vi "RT Loop - Analyze Acceleration_1.vi"(7 "testing":bool, 8 "error in (no error)":errorcluster, 9 "Acceleration RT FIFO In":T1, 10 "FPGA VI Reference Out":refnum<k20>, 11 "Message Queue":refnum<queue>) -> (1 "Acceleration RT FIFO Out":T1)   [LabVIEW 2017]
doc: "Read and analyze acceleration waveform data from FPGA via DMA FIFO. If the acceleration is over the limit, then send the acceleration waveform data to the Log Data Loop."
uses:
  <vilib>/rvi/interface/nirviMethod/nirviMethod.xnode
  <vilib>/FPGAPlugInAG/Dynamic/niLvFpga_ReadFifo_Dynamic.vi
  <vilib>/rvi/errors/niLvFpgaMergeErrorWithErrorCode.vi
  Globals/Global - All RT Loop Stop.vi
  Globals/Global - Configuration Options.vi
  UI Error Handlers/support/Logging/Logging.lvlib
  UI Error Handlers/support/Message Queue/Message Cluster.ctl
  UI Error Handlers/support/Message Queue/Message Queue.lvlib
  controls/Acceleration RT FIFO Reference.ctl
panel:
  out "x-y":u32
  out "G1 status":cluster{"G1 trigger":bool}
  out "G1 status.G1 trigger":bool
  out "sta":bool
  out "logical OR":bool
  in  "Data Rate (Hz)":dbl
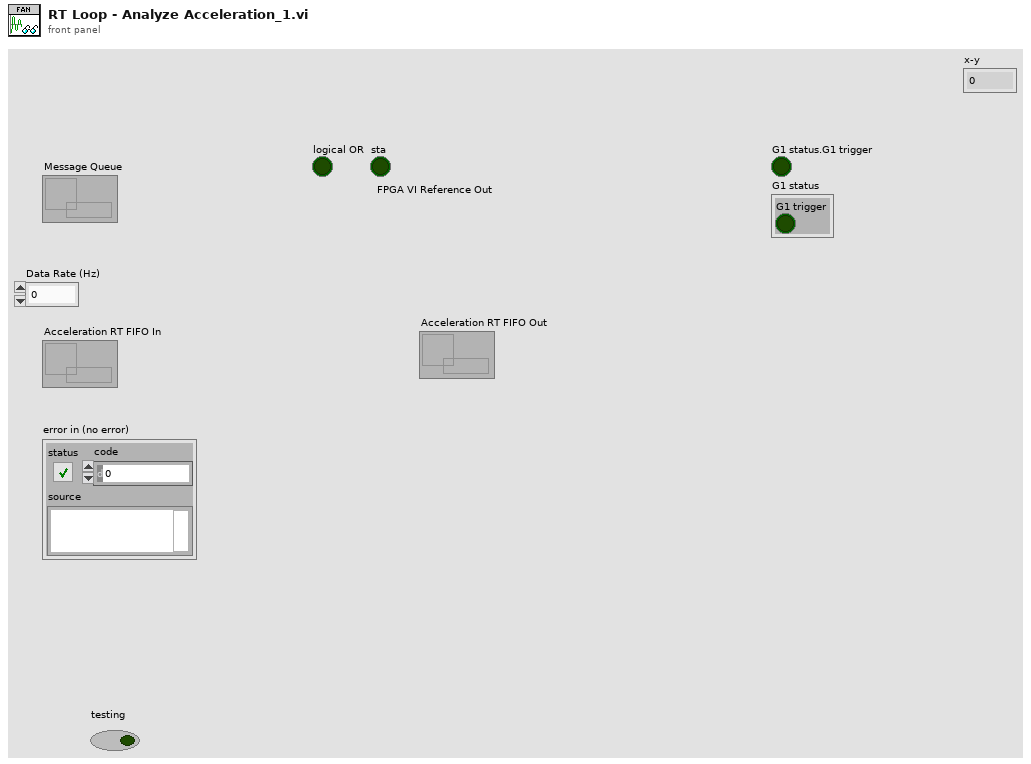
[diagram p1: front panel]
types:
  T1 = typedef "Acceleration RT FIFO Reference.ctl" = refnum<k33>
  T2 = cluster{"Tool data":cluster{"Number of teeth":sgl}, "Cutting data":cluster{"rpm":sgl}, "Limits":cluster{"Magnitude threshold":sgl, "Tolerance":sgl}, "G1 status":cluster{"G1 trigger":bool}}
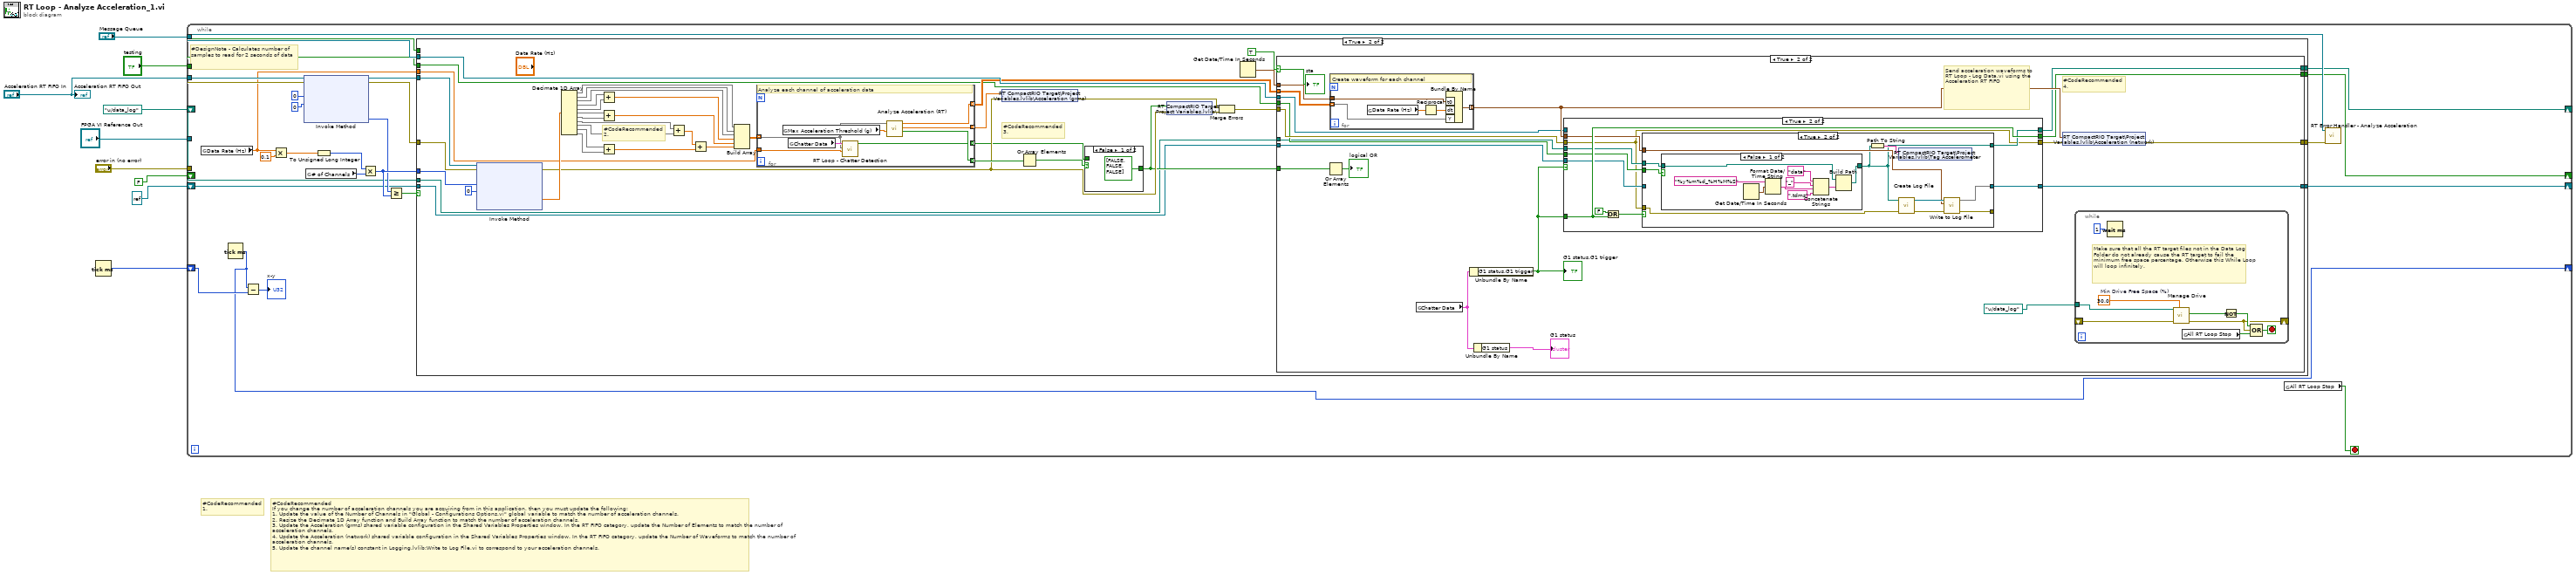
[diagram p0: block diagram]
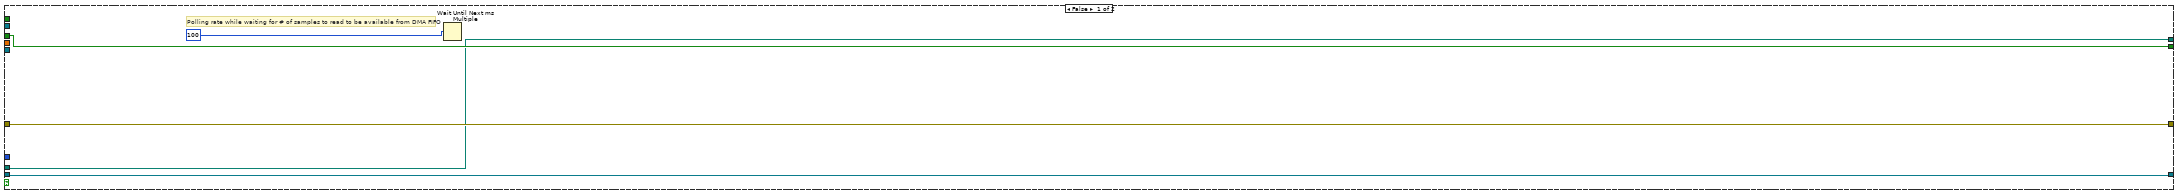
[diagram p2: hidden frame]
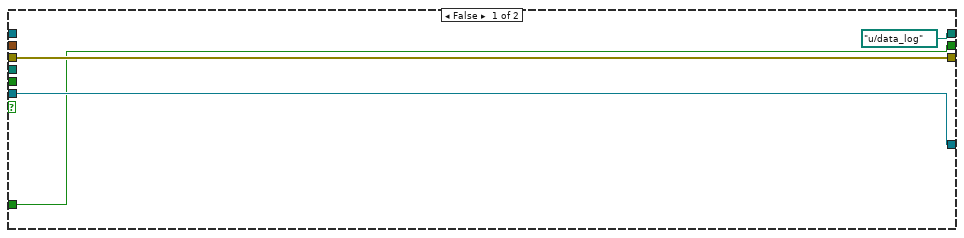
[diagram p5: hidden frame]
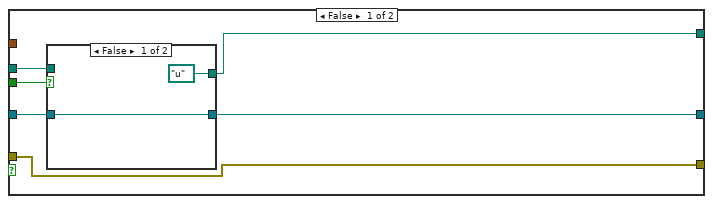
[diagram p6: hidden frame]
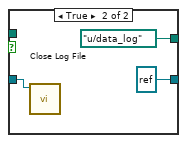
[diagram p7: hidden frame]
diagram:
  # "#CodeRecommended\n1."
  # "#CodeRecommended\nIf you change the number of acceleration channels you are acquiring from in this application, then you must update the following:\n1. Update the value of the Number of Channels in \"Global - Configurations Options.vi\" global variable to match the number of acceleration channels.\n2. Resize the Decimate 1D Array function and Build Array function to match the number of acceleration channels. \n3. Update the Acceleration (grms) shared variable configuration in the Shared Variables Properties window. In the RT FIFO category, update the Number of Elements to match the number of acceleration channels. \n4. Update the Acceleration (network) shared variable configuration in the Shared Variables Properties window. In the RT FIFO category, update the Number of Waveforms to match the number of acceleration channels.\n5. Update the channel name(s) constant in Logging.lvlib:Write to Log File.vi to correspond to your acceleration channels."
  n1 = Tick Count (ms)() -> (millisecond timer value=w1:u32)
  n2 = while {
    tunnel: "FPGA VI Reference Out" -> [w37]
    tunnel: "error in (no error)" -> [w36]
    tunnel: "Message Queue" -> [w29]
    tunnel: "Acceleration RT FIFO In" -> [w27]
    tunnel: "testing" -> [w19]
    shift-right: [w16] -> _
    shift-left: path "u:/data_log" ("AVI Path") -> [w15]
    shift-right: [w18] -> _
    shift-left: FALSE -> [w17]
    shift-right: [w14] -> _
    shift-left: refnum<k34> refnum ("Log File out") -> [w13]
    shift-right: [w11] -> _
    shift-left: w1 -> [w12]
    stop <- w30 stop-if-true
    # "#DesignNote - Calculates number of samples to read for 2 seconds of data"
    n3 = global read "Global - Configuration Options.vi" "Data Rate (Hz)"() -> (w21:dbl)
    n4 = Tick Count (ms)() -> (millisecond timer value=w11:u32)
    n5 = Subtract(x=w11, y=w12) -> (x-y=→"x-y":u32)
    n6 = Multiply(x=w21, y=0.1) -> (x*y=w25:dbl)
    n7 = xnode "Invoke Method"("FPGA VI Reference In"=w37, "error in"=w36, "Number of Elements"=u32 0, "Timeout (ms)"=0) -> ("FPGA VI Reference Out"=w33:refnum<k20>, "error out"=w32:errorcluster, "Elements Remaining"=w20:u32)  [unwired: 1 out]
    n8 = global read "Global - Configuration Options.vi" "# of Channels"() -> (w22:u32)
    n9 = To Unsigned Long Integer(number=w25) -> (unsigned 32bit integer=w24:u32)
    n10 = Multiply(x=w24, y=w22) -> (x*y=w23:u32)
    n11 = Greater Or Equal?(x=w20, y=w23) -> (x >= y?=w31:bool)
    n12 = case shown="True" w31 {
      tunnel: w33 -> [_ w85]
      tunnel: w32 -> [w42 w84]
      tunnel: [w42 w80] -> w28
      tunnel: w23 -> [_ w83]
      tunnel: w27 -> [_ w78]
      tunnel: w21 -> [_ w74]
      tunnel: w19 -> [_ _]
      tunnel: [w40 w66] -> w18
      tunnel: w17 -> [w40 w65]
      tunnel: [w39 w64] -> w16
      tunnel: w15 -> [w39 w63]
      tunnel: [w38 w62] -> w14
      tunnel: w13 -> [w38 w61]
      frame False {
        # "Polling rate while waiting for # of samples to read to be available from DMA FIFO"
        n13 = Wait Until Next ms Multiple(millisecond multiple=u32 100) -> ()  [unwired: 1 out]
      }
      frame True {
        # "#CodeRecommended\n3."
        # "#CodeRecommended\n2."
        n14 = xnode "Invoke Method"("FPGA VI Reference In"=w85, "error in"=w84, "Number of Elements"=w83, "Timeout (ms)"=0) -> ("error out"=w73:errorcluster, "Data"=w77:sgl[])  [unwired: 2 out]
        n15 = Decimate 1D Array(w77) -> (w58:sgl[], w57:sgl[], w56:sgl[], w55:sgl[], w54:sgl[], w52:sgl[], w51:sgl[], w50:sgl[], w49:sgl[], w48:sgl[], w47:sgl[])
        n16 = Add(x=w55, y=w54) -> (x+y=w53:sgl[])
        n17 = Add(x=w52, y=w51) -> (x+y=w43:sgl[])
        n18 = Add(x=w48, y=w47) -> (x+y=w45:sgl[])
        n19 = Add(x=w50, y=w49) -> (x+y=w46:sgl[])
        n20 = Add(x=w46, y=w45) -> (x+y=w44:sgl[])
        n21 = Build Array(w58, w57, w56, w53, w43, w44) -> (w59:sgl[][])
        n22 = for {
          tunnel: [w95] -> w79 mode=indexing
          tunnel: [w94] -> w76 mode=indexing
          tunnel: [w93] -> w75 mode=indexing
          tunnel: w74 -> [w91]
          tunnel: [w90] -> w68 mode=indexing
          tunnel: w59 -> [w88] mode=indexing
          # "Analyze each channel of acceleration data"
          n23 = global read "Global - Configuration Options.vi" "Max Acceleration Threshold (g)"() -> (w92:sgl)
          n24 = global read "Global - Configuration Options.vi" "Chatter Data"() -> (w89:T2)
          n25 = call "RT Loop - Chatter Detection.vi"("Data Rate (Hz)"=w91, "Acceleration Waveform (SGL)"=w88, "Chatter Data"=w89) -> ("Chatter?"=w90:bool)  [unwired: 8 in]
          n26 = call "Analyze Acceleration (RT).vi"("Max Instantaneous Acceleration (g)"=w92, "Acceleration Waveform (SGL)"=w88) -> ("Over Limit?"=w95:bool, "Acceleration (grms)"=w93:dbl, "Acceleration Waveform (DBL)"=w94:dbl[])  [unwired: 7 in]
        }
        n27 = shared-variable "RT CompactRIO Target\\Project Variables.lvlib\\Acceleration (grms)"(w75, error in=w73) -> (error out=w71:errorcluster)
        n28 = Or Array Elements(Boolean array=w79) -> (logical OR=w69:bool)
        n29 = case shown="False" w69 {
          tunnel: w68 -> [_ w87]
          tunnel: [bool[] [FALSE, FALSE, FALSE] ("Chatter?") w87] -> w67
          frame False {
          }
          frame True {
          }
        }
        n30 = shared-variable "RT CompactRIO Target\\Project Variables.lvlib\\Chatter?"(w67, error in=w73) -> (error out=w72:errorcluster)
        n31 = Merge Errors(w71, w72) -> (w70:errorcluster)
        n32 = Get Date/Time In Seconds() -> (seconds since 1Jan1904=w81:timestamp)
        n33 = case shown="True" TRUE {
          selector: TRUE -> [_ w111]
          tunnel: w81 -> [_ w119]
          tunnel: w70 -> [w99 w118]
          tunnel: [w99 w117] -> w80
          tunnel: w78 -> [_ w115]
          tunnel: w76 -> [_ w114]
          tunnel: w67 -> [_ w112]
          tunnel: [w98 w108] -> w66
          tunnel: w65 -> [w98 w107]
          tunnel: [w97 w106] -> w64
          tunnel: w63 -> [w97 w101]
          tunnel: [w96 w105] -> w62
          tunnel: w61 -> [w96 w104]
          frame False {
          }
          frame True {
            # "#CodeRecommended\n4."
            # "Send acceleration waveforms to RT Loop - Log Data.vi using the Acceleration RT FIFO"
            n34 = Or Array Elements(Boolean array=w112) -> (logical OR=→"logical OR":bool)
            n35 = for {
              tunnel: w114 -> [w178] mode=indexing
              tunnel: w119 -> [w177]
              tunnel: [w175] -> w116 mode=indexing
              # "Create waveform for each channel"
              n36 = global read "Global - Configuration Options.vi" "Data Rate (Hz)"() -> (w174:dbl)
              n37 = Reciprocal(x=w174) -> (1/x=w176:dbl)
              n38 = Bundle By Name("t0"=w177, "dt"=w176, "Y"=w178) -> (w175:waveform(dbl))  [unwired: 1 in]
            }
            n39 = global read "Global - Configuration Options.vi" "Chatter Data"() -> (w110:T2)
            n40 = Unbundle By Name(w110) -> ("G1 status.G1 trigger"=w102:bool)
            "G1 status.G1 trigger" <- w102
            n41 = Unbundle By Name(w110) -> ("G1 status"=→"G1 status":cluster{"G1 trigger":bool})
            n42 = case shown="True" w102 {
              tunnel: w118 -> [w132 w133]
              tunnel: w116 -> [_ w134]
              tunnel: w115 -> [_ _]
              tunnel: w102 -> [w130 w140]
              tunnel: [w130 w140] -> w108
              tunnel: w107 -> [_ w139]
              tunnel: [path "u:/data_log" ("AVI Path") w138] -> w106
              tunnel: w101 -> [_ w137]
              tunnel: [w131 w136] -> w105
              tunnel: w104 -> [w131 w135]
              tunnel: [w132 w133] -> w103
              frame False {
              }
              frame True {
                n43 = Or(x=FALSE, y=w140) -> (x .or. y?=w142:bool)
                n44 = case shown="True" w142 {
                  tunnel: w137 -> [w145 w163]
                  tunnel: [w148 w157] -> w138
                  tunnel: w139 -> [w146 w162]
                  tunnel: w135 -> [w147 _]
                  tunnel: w134 -> [_ w159]
                  tunnel: [w144 w156] -> w136
                  tunnel: w133 -> [w143 w155]
                  tunnel: [w143 w154] -> _
                  frame False {
                    n45 = case shown="False" w146 {
                      tunnel: [path "u:/" ("AVI Path") path "u:/data_log" ("AVI Path")] -> w148
                      tunnel: w147 -> [w149 w152]
                      tunnel: w145 -> [_ _]
                      tunnel: [w149 refnum<k34> refnum ("Log File out")] -> w144
                      frame False {
                      }
                      frame True {
                        n46 = call "Close Log File.vi"("tdms file"=w152) -> ()  [unwired: 10 in, 1 out]
                      }
                    }
                  }
                  frame True {
                    n47 = case shown="False" w162 {
                      tunnel: w163 -> [w165 w173]
                      tunnel: [w164 w173] -> w157
                      frame False {
                        n48 = Get Date/Time In Seconds() -> (seconds since 1Jan1904=w168:timestamp)
                        n49 = Format Date/Time String(time format string (%c)="%y%m%d_%H%M%S", seconds (now)=w168) -> (date/time string=w171:string)  [unwired: 1 out]
                        n50 = Concatenate Strings("data" ("string"), "_" ("string"), w171, ".tdms" ("string")) -> (w166:string)
                        n51 = Build Path(base path=w165, name or relative path=w166) -> (appended path=w164:path)
                      }
                      frame True {
                      }
                    }
                    n52 = Path To String(path=w157) -> (string=w158:string)
                    n53 = shared-variable "RT CompactRIO Target\\Project Variables.lvlib\\Tag Accelerometer"(w158) -> ()  [unwired: 1 in, 1 out]
                    n54 = call "Create Log File.vi"("error in (no error)"=w155, "Acceleration Exceeded Log Folder"=w157) -> ("error out"=w161:errorcluster, "Log File out"=w160:refnum<k34>)  [unwired: 8 in]
                    n55 = call "Write to Log File.vi"("error in (no error)"=w161, "Array of Waveforms"=w159, "Log File in"=w160) -> ("error out"=w154:errorcluster, 3:w156)  [unwired: 7 in]
                  }
                }
              }
            }
            n56 = shared-variable "RT CompactRIO Target\\Project Variables.lvlib\\Acceleration (network)"(w116, error in=w103) -> (error out=w117:errorcluster)
            n57 = while {
              shift-right: [w123] -> _
              shift-left: _ -> [w124]
              tunnel: path "u:/data_log" ("AVI Path") -> [w121]
              stop <- w128 stop-if-true
              w122 = 30.0  # Min Drive Free Space (%)
              # "Make sure that all the RT target files not in the Data Log Folder do not already cause the RT target to fail the minimum free space percentage. Otherwise this While Loop will loop infinitely."
              n58 = Wait (ms)(milliseconds to wait=u32 1) -> ()  [unwired: 1 out]
              n59 = call "Manage Drive.vi"("Min Drive Free Space (%)"=w122, "error in"=w124, "Data Folder"=w121) -> ("error out"=w123:errorcluster, "Drive Space Below Limit"=w120:bool)  [unwired: 6 in, 1 out]
              n60 = global read "Global - All RT Loop Stop.vi" "All RT Loop Stop"() -> (w125:bool)
              n61 = Not(x=w120) -> (.not. x?=w127:bool)
              n62 = Compound Arithmetic op=OR(w127, w123, w125) -> (w128:bool)
            }
            "sta" <- w111
          }
        }
      }
    }
    n63 = global read "Global - All RT Loop Stop.vi" "All RT Loop Stop"() -> (w30:bool)
    n64 = call "RT Error Handler - Analyze Acceleration.vi"("error in (no error)"=w28, "Message Queue"=w29) -> ()  [unwired: 9 in, 1 out]
  }
  "Acceleration RT FIFO Out" <- "Acceleration RT FIFO In"
